vi "New Subscription Request.vi"(8 "Subscription Policy":T1, 10 "Type":variant, 11 "Datum Name":string) -> (3 "SubscriptionRequest":refnum<class "SubscriptionRequest.lvclass">)   [LabVIEW 2017, in "IMediator.lvlib" / "SubscriptionRequest.lvclass"]
doc: "Use \"Pack Subscription Request\" (Same thing, new name)"
uses:
  SubscriptionRequest.lvclass
  ISubscriptionPolicy/ISubscriptionPolicy Reference.ctl
  ISubscriptionPolicy/ISubscriptionPolicy.lvclass
  SubscriptionRequest.lvclass/SubscriptionRequest.ctl
panel:
  # "Use Pack Subscription Request"
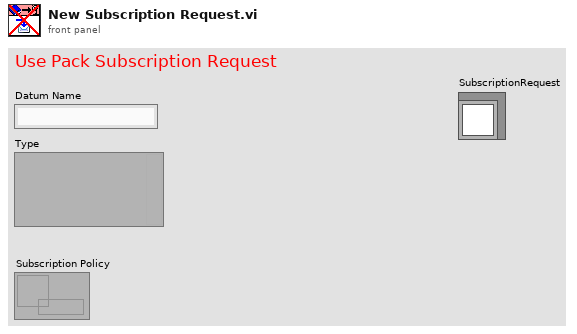
[diagram p1: front panel]
types:
  T1 = typedef "IMediator.lvlib/ISubscriptionPolicy.lvclass/ISubscriptionPolicy Reference.ctl" = refnum<data-value>
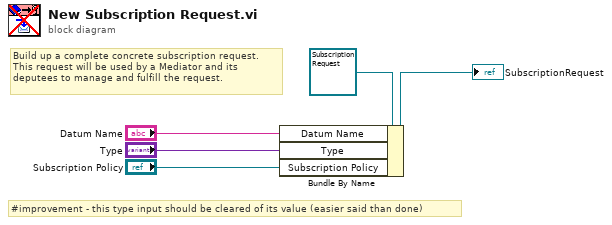
[diagram p0: block diagram]
diagram:
  # "Build up a complete concrete subscription request.\nThis request will be used by a Mediator and its\ndeputees to manage and fulfill the request."
  # "#improvement - this type input should be cleared of its value (easier said than done)"
  n1 = Bundle By Name(cluster=refnum<class "SubscriptionRequest.lvclass"> refnum ("SubscriptionRequest in"), "Datum Name"="Datum Name", "Type"="Type", "Subscription Policy"="Subscription Policy") -> (→"SubscriptionRequest":refnum<class "SubscriptionRequest.lvclass">)
